vi "01 - Calling NET Simple.vi"() -> ()   [LabVIEW 2021]
uses:
  <vilib>/JDP Science/JSONtext/JSONtext.lvlib
  <vilib>/Utility/sysdir.llb/System Directory Type.ctl
panel:
  out "File Watcher Event Data\n<JSON>":string
  out "error out":errorcluster
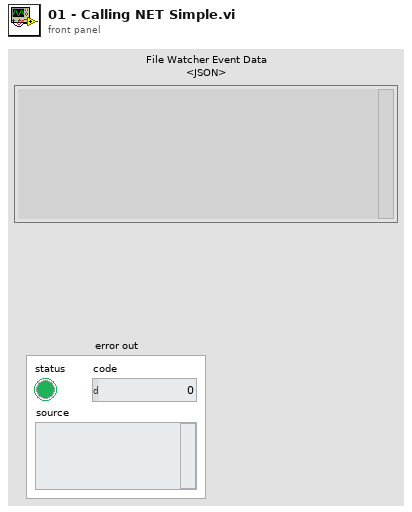
[diagram p1: front panel]
types:
  T1 = typedef "System Directory Type.ctl" = i32
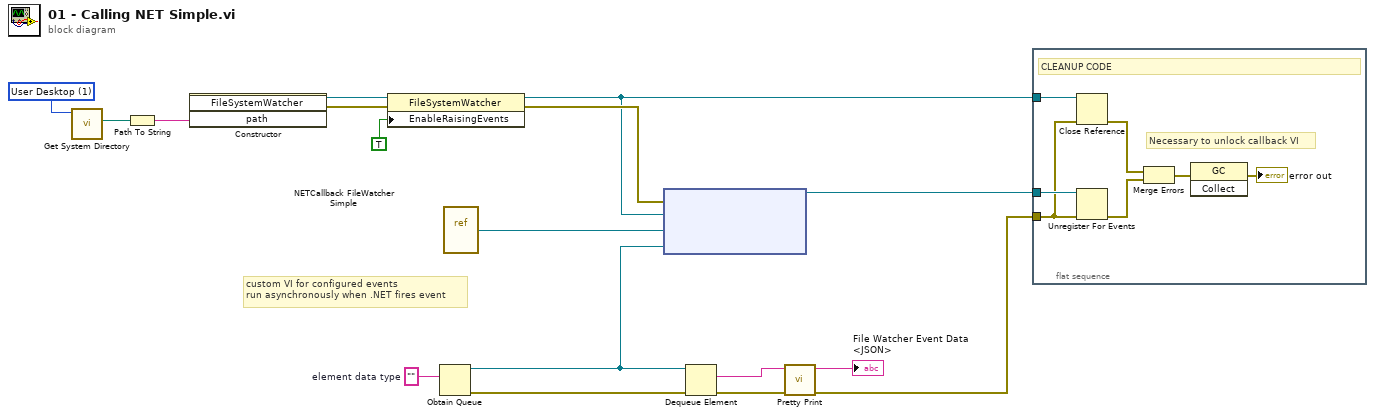
[diagram p0: block diagram]
diagram:
  w14 = ""  # element data type
  w9 = T1 1 items=["User Home"=0, "User Desktop"=1, "User Documents"=2, "User Application Data"=3, "User Preferences"=4, "User Temporary"=5, "Public Documents"=6, "Public Application Data"=7, "Public Preferences"=8, "Public Cache"=13, "System Core Libraries"=9, "System Installed Libraries"=10, "Application Files"=11, "Boot Volume Root"=12] ("system directory type")
  # "custom VI for configured events\nrun asynchronously when .NET fires event"
  n1 = call <vilib>:"Get System Directory.vi"("system directory type"=w9) -> ("system directory"=w8:path)  [unwired: 10 in]
  n2 = Path To String(path=w8) -> (string=w15:string)
  n3 = constructor class="FileSystemWatcher"("path"=w15) -> (reference out=w11:refnum<k24>, error out=w16:errorcluster)  [unwired: 3 in, 2 out]
  n4 = property class="FileSystemWatcher"(reference=w11, error in=w16, "EnableRaisingEvents"=TRUE) -> (reference out=w13:refnum<k24>, error out=w17:errorcluster)
  n5 = Obtain Queue(element data type=w14) -> (queue out=w3:refnum<queue>, error out=w2:errorcluster)  [unwired: 4 in, 1 out]
  n6 = vi-ref "NETCallback FileWatcher Simple.vi"() -> (w4:refnum<vi>)
  n7 = node(w17, w13, w4, w3) -> (w12:refnum<k27>)  [unwired: 1 in, 1 out]
  n8 = Dequeue Element(queue=w3, error in (no error)=w2) -> (element=w7:string, error out=w5:errorcluster)  [unwired: 1 in, 2 out]
  n9 = call <vilib>:"Pretty Print.vi"("error in (no error)"=w5, "JSON"=w7) -> ("error out"=w1:errorcluster, "<JSON>"=→"File Watcher Event Data\n<JSON>":string)  [unwired: 7 in, 1 out]
  n10 = flat-sequence {
    tunnel: w13 -> [w20]
    tunnel: w12 -> [w19]
    tunnel: w1 -> [w18]
    frame #0 {
      # "Necessary to unlock callback VI"
      # "CLEANUP CODE"
      n11 = Close Reference(reference=w20, error in (no error)=w18) -> (error out=w22:errorcluster)
      n12 = Unregister For Events(event registration refnum=w19, error in=w18) -> (error out=w21:errorcluster)
      n13 = Merge Errors(w22, w21) -> (w23:errorcluster)
      n14 = invoke class="GC" method="Collect"(error in=w23) -> (error out=→"error out":errorcluster)  [unwired: 2 in, 2 out]
    }
  }
